vi "Core_Put Notifier.vi"(8 "error in (no error)":errorcluster, 9 "Data":variant, 10 "Notifier Type":T1=enum."Receive Message", 11 "HSMS Class in":refnum<class "HSMS Class.lvclass">) -> (0 "error out":errorcluster, 3 "HSMS Class out":refnum<class "HSMS Class.lvclass">)   [LabVIEW 2020, in "SECS Communication.lvlib" / "HSMS Class.lvclass"]
uses:
  HSMS Class.lvclass
  Notifier Type.ctl
  Notifier Data.ctl
  HSMS Class.lvclass/HSMS Class.ctl
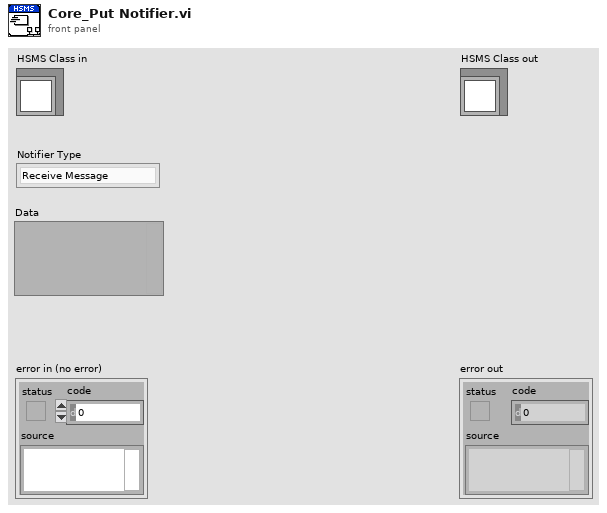
[diagram p1: front panel]
types:
  T1 = typedef "SECS Communication.lvlib/HSMS Class.lvclass/Notifier Type.ctl" = enum16{"TCPIP Connect", "TCPIP Disconnect", "Receive Message", "Send Message", "T3 Timeout", "T6 Timeout", "T7 Timeout", "Error", "Stop"}
  T2 = typedef "SECS Communication.lvlib/HSMS Class.lvclass/Notifier Data.ctl" = cluster{"Notifier Type":T1, "Data":variant, "Time":timestamp}
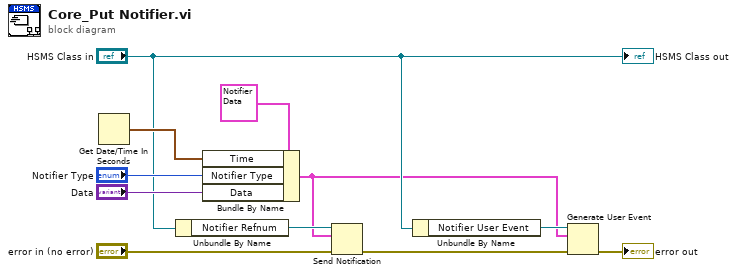
[diagram p0: block diagram]
diagram:
  n1 = Get Date/Time In Seconds() -> (seconds since 1Jan1904=w6:timestamp)
  n2 = Unbundle By Name("HSMS Class in") -> ("Notifier Refnum"=w11:refnum<notifier>)
  n3 = Bundle By Name(cluster=T2 {"Notifier Type"=enum."Send Message", "Data"=variant, "Time"=timestamp(0 s since 1904-01-01)} ("notification"), "Time"=w6, "Notifier Type"="Notifier Type", "Data"="Data") -> (w2:T2)
  n4 = Send Notification(notification=w2, notifier=w11, error in (no error)="error in (no error)") -> (error out=w4:errorcluster)  [unwired: 1 out]
  n5 = Unbundle By Name("HSMS Class in") -> ("Notifier User Event"=w5:refnum<user-event>)
  n6 = Generate User Event(user event=w5, event data cluster=w2, error in=w4) -> (error out=→"error out":errorcluster)  [unwired: 1 in, 1 out]
  "HSMS Class out" <- "HSMS Class in"
